vi "Read Key.vi"(8 "Error In":errorcluster, 11 "Known Host In":refnum<class "KnownHost.lvclass">) -> (0 "Error Out":errorcluster, 2 "Key":u8[](array[numeric]), 3 "Known Host Out":refnum<class "KnownHost.lvclass">)   [LabVIEW 2017, in "Toolkit.lvlib" / "KnownHost.lvclass"]
uses:
  KnownHost.lvclass
  KnownHost.lvclass/KnownHost.ctl
  Toolkit.lvlib
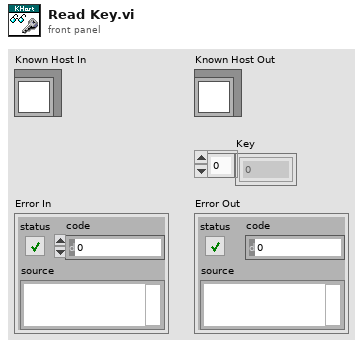
[diagram p1: front panel]
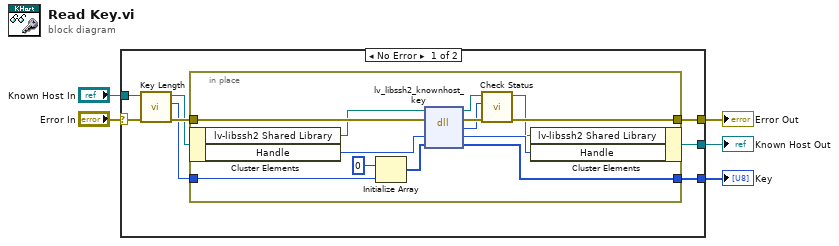
[diagram p0: block diagram]
diagram:
  n1 = case shown="No Error" "Error In" {
    selector: "Error In" -> [w12 w28]
    tunnel: [w13 w28] -> w4
    tunnel: "Known Host In" -> [w10 w27]
    tunnel: [w7 w27] -> w2
    tunnel: [w6 _] -> w1
    frame No Error {
      n2 = call "Key Length.vi"("Error In"=w12, "Known Host In"=w10) -> ("Error Out"=w11:errorcluster, "Length"=w8:u64, "Known Host Out"=w9:refnum<class "KnownHost.lvclass">)  [unwired: 7 in]
      n3 = in-place {
        in-place-border: w11 -> [w26]
        in-place-border: [w23] -> w13
        in-place-border: w8 -> [w18]
        in-place-border: [w14] -> w6
        n4 = in-place-cluster #1(w9) -> ("lv-libssh2 Shared Library"=w16:path, "Handle"=w15:u64)
        n5 = Initialize Array(u8 0, w18) -> (w17:u8[])
        n6 = dll-call lib="lv-libssh2.*" fn="lv_libssh2_knownhost_key"(path in=w16, error in=w26, "handle"=w15, "buffer"=w17) -> (path out=w22:path, error out=w24:errorcluster, "status"=w20:i32, "handle"=w25:u64, "buffer"=w14:u8[])  [unwired: 1 in]
        n7 = call "Check Status.vi"("Error In"=w24, "Status"=w20, "lv-libssh2 Shared Library In"=w22) -> ("Error Out"=w23:errorcluster, "lv-libssh2 Shared Library Out"=w21:path)  [unwired: 7 in]
        n8 = in-place-cluster #1("lv-libssh2 Shared Library"=w21, "Handle"=w25) -> (w7:refnum<class "KnownHost.lvclass">)
      }
    }
    frame Error {
    }
  }
  "Error Out" <- w4
  "Known Host Out" <- w2
  "Key" <- w1
